vi "BuildQueryString.vi"(10 "QueryStringItems":T1(array[cluster]), 11 "QueryStringIn":string) -> (3 "QueryStringOut":string)   [LabVIEW 2015]
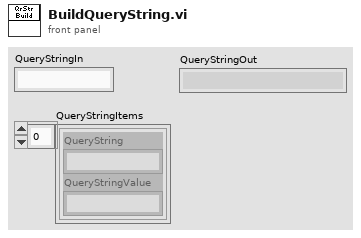
[diagram p1: front panel]
types:
  T1 = cluster{"QueryString":string, "QueryStringValue":string}[]
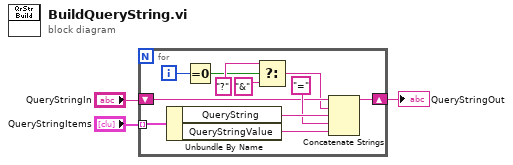
[diagram p0: block diagram]
diagram:
  n1 = for {
    tunnel: "QueryStringItems" -> [w13] mode=indexing
    shift-right: [w14] -> w2
    shift-left: "QueryStringIn" -> [w5]
    i -> [w7]
    n2 = Unbundle By Name(w13) -> ("QueryString"=w10:string, "QueryStringValue"=w8:string)
    n3 = Equal To 0?(x=w7) -> (x = 0?=w6:bool)
    n4 = Select(t="?", s=w6, f="&") -> (s? t:f=w4:string)
    n5 = Concatenate Strings(w5, w4, w10, "=", w8) -> (w14:string)
  }
  "QueryStringOut" <- w2
